vi "global reset.vi"(8 "error in (no error)":errorcluster, 11 "identifier":string) -> (0 "error out":errorcluster, 2 "function return":u32, 3 "identifier out":string)   [LabVIEW 2015, in "XGL_DPP.lvlib"]
doc: "EXTERN DECLSPEC unsigned int CALL_CONV global_reset(char* identifier);"
uses:
  XGL_DPP.lvlib
  D:/Scanning Software_Demokritos_2015_v6/libs/XGL_DPP.dll
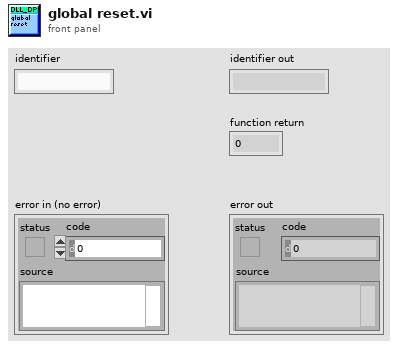
[diagram p1: front panel]
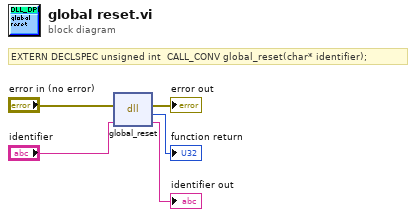
[diagram p0: block diagram]
diagram:
  # "EXTERN DECLSPEC unsigned int  CALL_CONV global_reset(char* identifier);"
  n1 = dll-call lib="D:/Scanning Software_Demokritos_2015_v6/libs/XGL_DPP.*" fn="global_reset"(error in="error in (no error)", "identifier"="identifier") -> (error out=→"error out":errorcluster, "return type"=→"function return":u32, "identifier"=→"identifier out":string)  [unwired: 2 in, 1 out]
